vi "booleanos.vi"() -> ()   [LabVIEW 2020]
panel:
  out "CA":bool
  out "NOT":bool
  out "XOR":bool
  out "OR":bool
  in  "Boton2":bool
  out "AND":bool
  in  "Boton1":bool
  # "Booleanos"
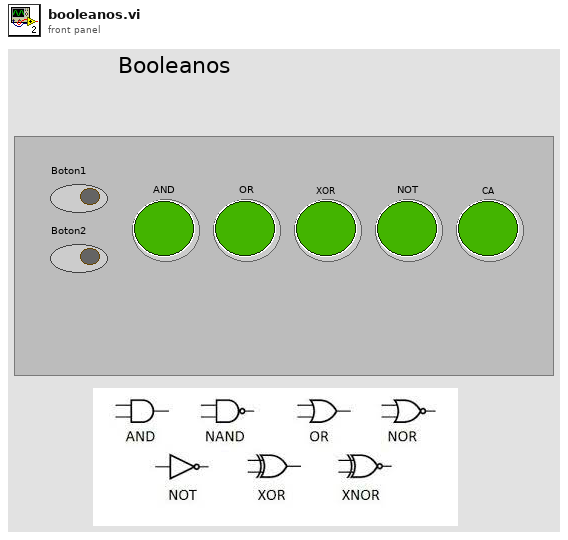
[diagram p1: front panel]
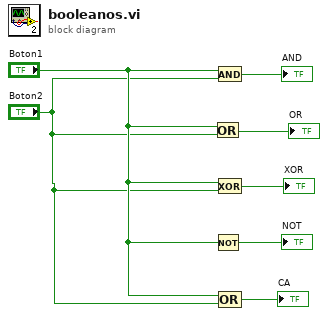
[diagram p0: block diagram]
diagram:
  n1 = Or(x="Boton1", y="Boton2") -> (x .or. y?=→"OR":bool)
  n2 = Not(x="Boton1") -> (.not. x?=→"NOT":bool)
  n3 = And(x="Boton1", y="Boton2") -> (x .and. y?=→"AND":bool)
  n4 = Exclusive Or(1:"Boton2", 2:"Boton1") -> (0:→"XOR":bool)
  n5 = Compound Arithmetic op=OR("Boton1", "Boton2") -> (→"CA":bool)
